vi "LVCAM Create Nest.vi"(9 "Alias":string, 10 "Nest Actor":refnum<class "LVCAM.lvclass">, 11 "LVCAM Create Nest Msg in":refnum<class "LVCAM Create Nest Msg.lvclass">) -> (0 "error out":errorcluster, 3 "LVCAM Create Nest Msg out":refnum<class "LVCAM Create Nest Msg.lvclass">)   [LabVIEW 2021, in "LVCAM Create Nest.lvlib" / "LVCAM Create Nest Msg.lvclass"]
uses:
  LVCAM Create Nest Msg.lvclass
  LVCAM/LVCAM/LVCAM.lvclass
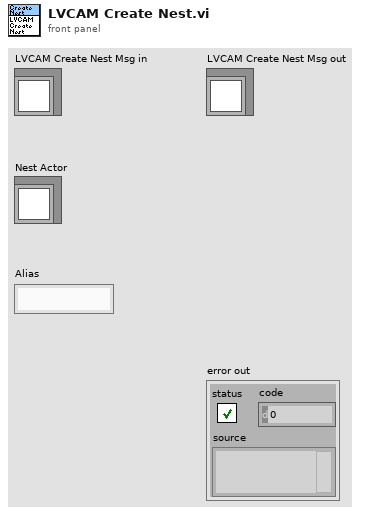
[diagram p1: front panel]
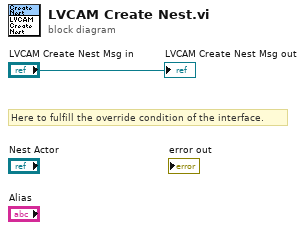
[diagram p0: block diagram]
diagram:
  # "Here to fulfill the override condition of the interface."
  "LVCAM Create Nest Msg out" <- "LVCAM Create Nest Msg in"
